vi "Write AINames.vi"(8 "error in (no error)":errorcluster, 10 "ALRNames":string[][](array[string]), 11 "AI in":T1) -> (0 "error out":errorcluster, 3 "AI out":T1)   [LabVIEW 2019, in "Inputs.lvlib"]
uses:
  Inputs.lvlib
  Ctl/AI.ctl
  Ctl/AI short.ctl
  Ctl/Parameter State.ctl
panel:
  # "Analog parameters"
  # "Description of analog parameters"
  # "Analog parameters"
  # "Description of analog parameters"
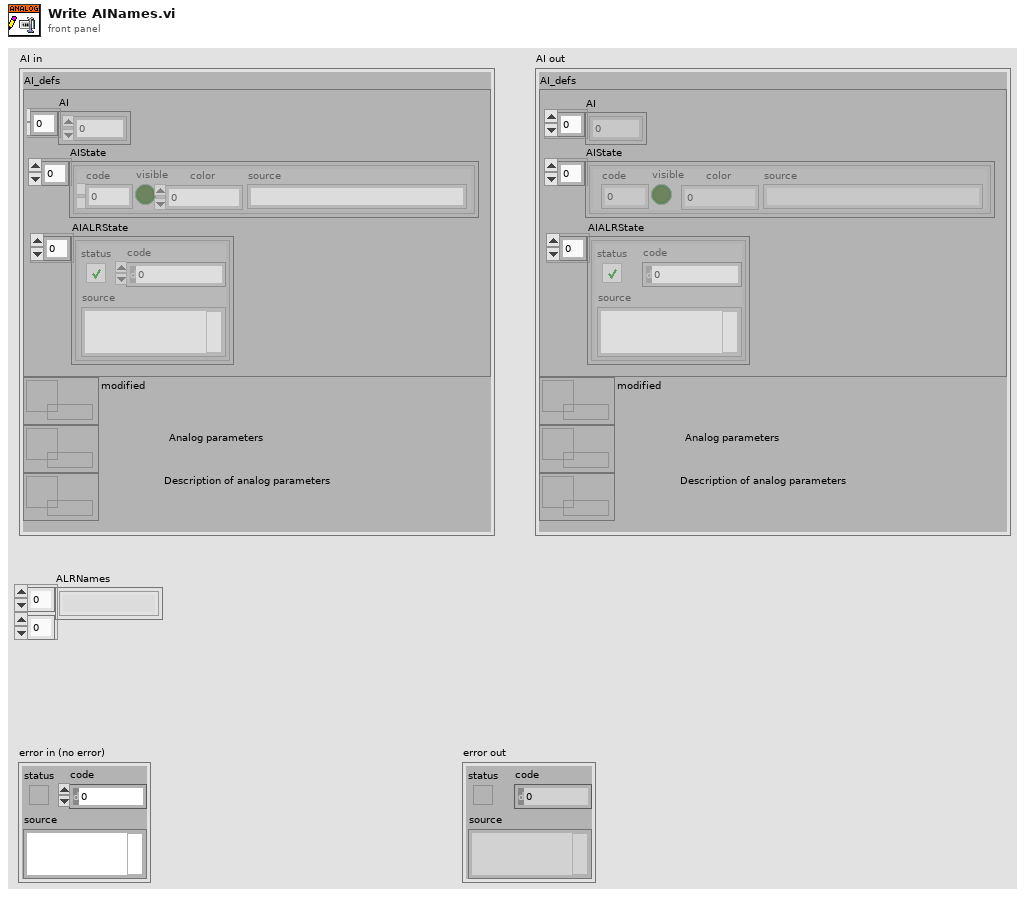
[diagram p1: front panel]
types:
  T1 = typedef "Inputs.lvlib/AI.ctl" = cluster{"AI_defs":T2, "modified":refnum<data-value>, "AIP":refnum<data-value>, "AINames":refnum<data-value>}
  T2 = typedef "Inputs.lvlib/AI short.ctl" = cluster{"AI":dbl[], "AIState":T3[], "AIALRState":errorcluster[]}
  T3 = typedef "Inputs.lvlib/Parameter State.ctl" = cluster{"code":i32, "visible":bool, "color":u32, "source":string}
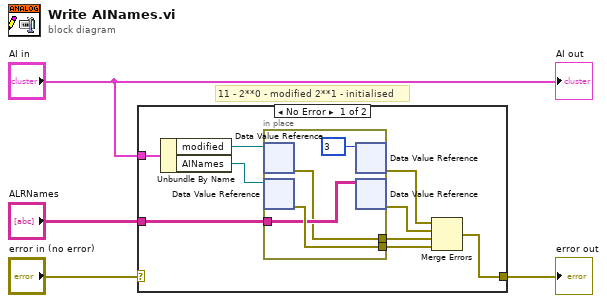
[diagram p0: block diagram]
diagram:
  # "11 - 2**0 - modified 2**1 - initialised"
  n1 = case shown="No Error" "error in (no error)" {
    selector: "error in (no error)" -> [_ w18]
    tunnel: [w10 w18] -> w1
    tunnel: "AI in" -> [w5 _]
    tunnel: "ALRNames" -> [w11 _]
    frame No Error {
      n2 = Unbundle By Name(w5) -> ("modified"=w9:refnum<data-value>, "AINames"=w13:refnum<data-value>)
      n3 = in-place {
        in-place-border: w11 -> [w16]
        in-place-border: [w17] -> w7
        in-place-border: [w15] -> w6
        n4 = in-place-dvr #1(w9) -> (w15:errorcluster)  [unwired: 1 out]
        n5 = in-place-dvr #2(w13) -> (w17:errorcluster)  [unwired: 1 out]
        n6 = in-place-dvr #1(u8 3 ("data value")) -> (w8:errorcluster)  [unwired: 1 out]
        n7 = in-place-dvr #2(w16) -> (w12:errorcluster)  [unwired: 1 out]
      }
      n8 = Merge Errors(w8, w12, w6, w7) -> (w10:errorcluster)
    }
    frame Error {
    }
  }
  "error out" <- w1
  "AI out" <- "AI in"
